vi "Introspection Core.vi"(8 "error in (no error)":errorcluster, 11 "CS++PVMonitor in":refnum<class "CS++PVMonitor.lvclass">) -> (0 "error out":errorcluster, 2 "CS++Messages":refnum<class "Message.lvclass">[](array[class]), 3 "CS++PVMonitor out":refnum<class "CS++PVMonitor.lvclass">)   [LabVIEW 2014, in "CS++PVMonitor.lvlib" / "CS++PVMonitor.lvclass"]
doc: "This vi delivers a list with all messages this actor reacts to. \n\nNote that all inherited classes have to overwrite it."
uses:
  CS++PVMonitor.lvclass
  <vilib>/ActorFramework/Message/Message.lvclass
  CS++BaseActor/CS++BaseActor.lvclass
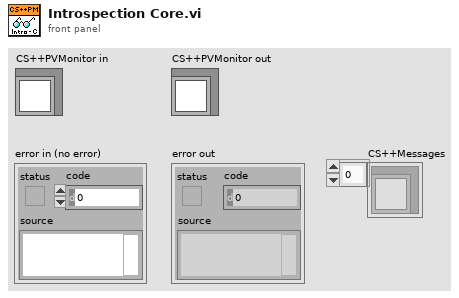
[diagram p1: front panel]
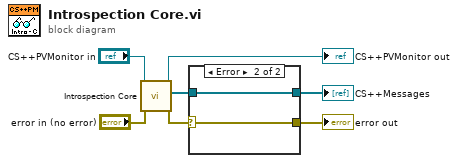
[diagram p0: block diagram]
diagram:
  n1 = call-parent "Introspection Core.vi"("error in (no error)"="error in (no error)", "CS++BaseActor in"="CS++PVMonitor in") -> ("error out"=w4:errorcluster, "CS++Messages"=w2:refnum<class "Message.lvclass">[], "CS++BaseActor out"=→"CS++PVMonitor out":refnum<class "CS++PVMonitor.lvclass">)  [unwired: 7 in]
  n2 = case shown="Error" w4 {
    selector: w4 -> [w9 w11]
    tunnel: [w9 w11] -> w3
    tunnel: w2 -> [w8 w10]
    tunnel: [w8 w10] -> w1
    frame No Error {
    }
    frame Error {
    }
  }
  "error out" <- w3
  "CS++Messages" <- w1
